vi "Construct DMD Intensity Coefficients (SubVI).vi"(7 "DMD #":enum16{"DMD1", "DMD2"}(ring), 8 "Number of Rows Processed":refnum<vi>, 11 "Image Size in":T1={"Height"=3072, "Width"=3200}) -> ()   [LabVIEW 2015]
uses:
  Controls (HOST)/Image Size.ctl
  <vilib>/Utility/file.llb/Read Delimited Spreadsheet (DBL).vi
  <vilib>/imath/engines/lvmath2/RunTimeEngine/Managers/WorkSpace/UID Generator.vi
  <vilib>/imath/engines/lvmath2/RunTimeEngine/RunTimeType/NIMS_RunTimeType_From StrictType (excl LVString).vi
  <instcachedir>/0/NIMS_RunTimeType_From StrictType (excl LVString)_EB1C38A9BC5048DA9ABDA8F781E54D21.lvgen/NIMS_RunTimeType_From StrictType (excl LVString)_EB1C38A9BC5048DA9ABDA8F781E54D21_031.vi
  <vilib>/imath/engines/lvmath2/RunTimeEngine/Struct/NIMS_StructSetField.vi
  <vilib>/imath/engines/lvmath2/RunTimeEngine/Struct/NIMS_StructGetField.vi
  <vilib>/imath/engines/lvmath2/RunTimeEngine/RunTimeType/NIMS_RunTimeType_To Numeric.vi
  <instcachedir>/0/NIMS_RunTimeType_To Numeric_B134FEC7BFC54ED5998F4CFD2EE98288.lvgen/NIMS_RunTimeType_To Numeric_B134FEC7BFC54ED5998F4CFD2EE98288_008.vi
  <instcachedir>/0/NIMS_RunTimeType_From StrictType (excl LVString)_EB1C38A9BC5048DA9ABDA8F781E54D21.lvgen/NIMS_RunTimeType_From StrictType (excl LVString)_EB1C38A9BC5048DA9ABDA8F781E54D21_000.vi
  <vilib>/imath/engines/lvmath2/RunTimeEngine/LocalVariableDefStatement/MC_LocalVariableDefStatement_Display.vi
  <vilib>/imath/engines/lvmath2/RunTimeEngine/Managers/SymbolTable/Clear UID.vi
  <vilib>/imath/engines/lvmath2/RunTimeEngine/NodeEndStatement/NIMS_NodeEndStatement_Output.vi
  <instcachedir>/0/NIMS_NodeEndStatement_Output_53EC0D466D134D7ABD903AC30B43404B.lvgen/NIMS_NodeEndStatement_Output_53EC0D466D134D7ABD903AC30B43404B_001.vi
  <vilib>/imath/engines/lvmath2/RunTimeEngine/ErrorHandling/NIMS_Finalize Error.vi
  <vilib>/Utility/file.llb/Write Delimited Spreadsheet (DBL).vi
  <vilib>/imath/engines/lvmath2/RunTimeEngine/Managers/SymbolTable/NIMS_WorkSpace.lvlib
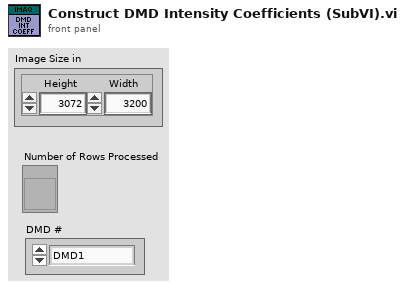
[diagram p1: front panel]
types:
  T1 = typedef "Image Size.ctl" = cluster{"Height":u16, "Width":u16}
  T2 = typedef "DMD 2 Calibration Parameters.ctl" = cluster{"xm1":dbl, "ym1":dbl, "xm2":dbl, "ym2":dbl, "xoff":dbl, "yoff":dbl}
  T3 = typedef "DMD 1 Calibration Parameters.ctl" = cluster{"xm1":dbl, "ym1":dbl, "xm2":dbl, "ym2":dbl, "xoff":dbl, "yoff":dbl}
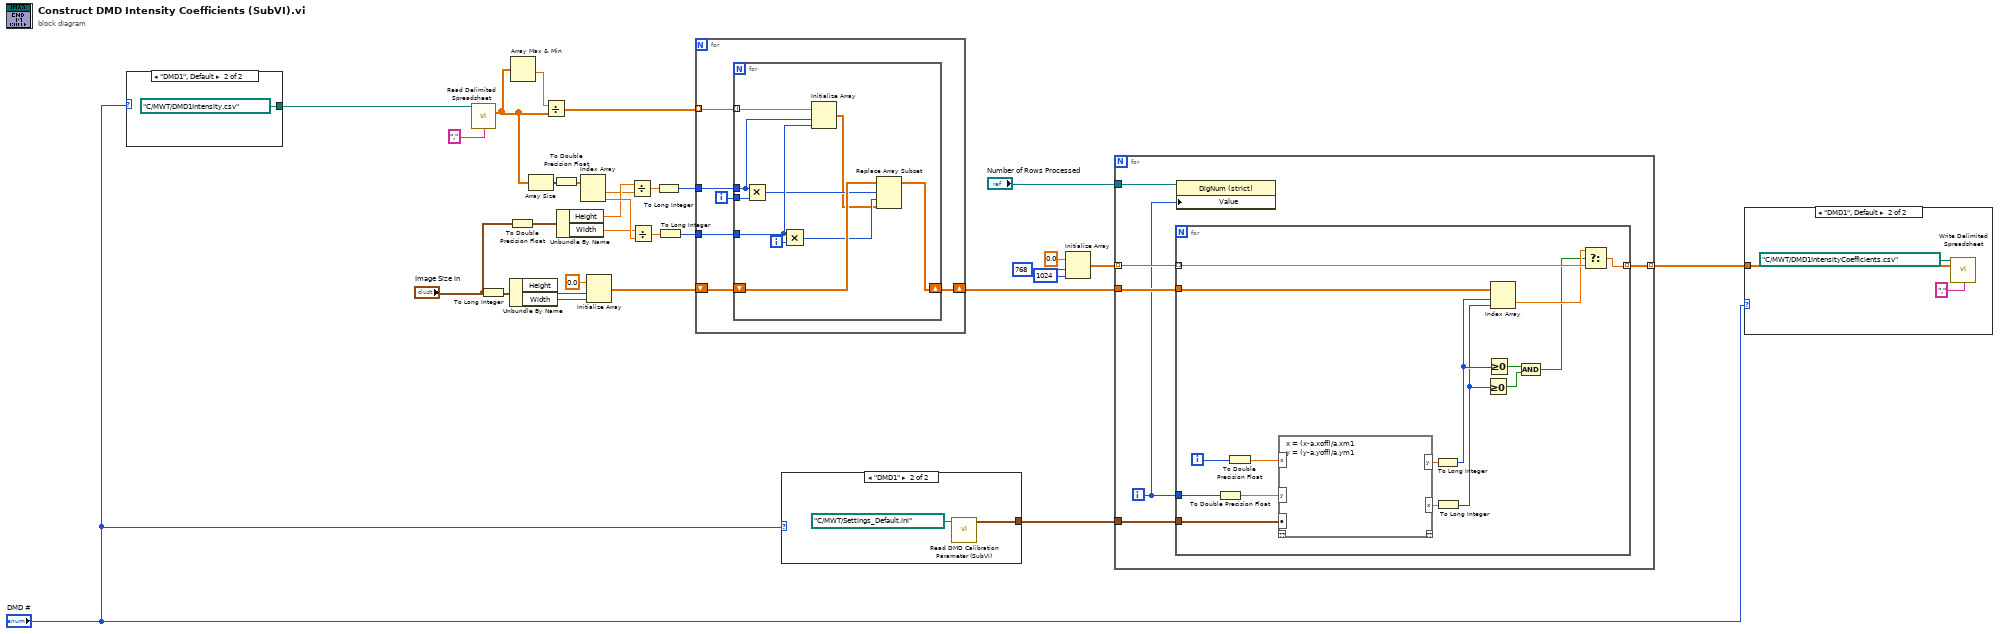
[diagram p0: block diagram]
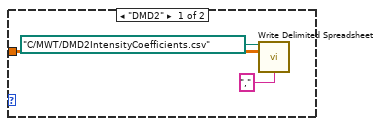
[diagram p2: hidden frame]
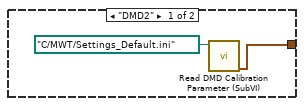
[diagram p3: hidden frame]
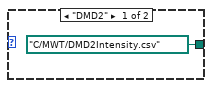
[diagram p4: hidden frame]
diagram:
  n1 = case shown="\"DMD1\", Default" "DMD #" {
    tunnel: [path "C:/MWT/DMD2Intensity.csv" ("file path (dialog if empty)") path "C:/MWT/DMD1Intensity.csv" ("file path (dialog if empty)")] -> w4
    frame "DMD2" {
    }
    frame "DMD1", Default {
    }
  }
  n2 = call-poly <vilib>:"Read Delimited Spreadsheet.vi"("file path (dialog if empty)"=w4, "delimiter (\\t)"="," ("delimiter (\\t)")) -> ("all rows"=w10:dbl[][])  [unwired: 8 in, 5 out]
  n3 = To Long Integer(number="Image Size in") -> (32bit integer=w9:cluster{"Height":i32, "Width":i32})
  n4 = To Double Precision Float(number="Image Size in") -> (double precision float=w15:cluster{"Height":dbl, "Width":dbl})
  n5 = Unbundle By Name(w9) -> ("Height"=w6:i32, "Width"=w7:i32)
  n6 = Array Max & Min(array=w10) -> (min value=w5:dbl)  [unwired: 3 out]
  n7 = Array Size(array=w10) -> (size(s)=w11:i32[])
  n8 = Divide(x=w5, y=w10) -> (x/y=w13:dbl[][])
  n9 = To Double Precision Float(number=w11) -> (double precision float=w14:dbl[])
  n10 = Unbundle By Name(w15) -> ("Height"=w17:dbl, "Width"=w18:dbl)
  n11 = Index Array(array=w14) -> (element #1=w16:dbl, element #2=w19:dbl)  [unwired: 2 in]
  n12 = Initialize Array(0.0 ("element"), w6, w7) -> (w12:dbl[][])
  n13 = Divide(x=w17, y=w16) -> (x/y=w20:dbl)
  n14 = Divide(x=w18, y=w19) -> (x/y=w21:dbl)
  n15 = To Long Integer(number=w20) -> (32bit integer=w22:i32)
  n16 = To Long Integer(number=w21) -> (32bit integer=w23:i32)
  n17 = for {
    shift-right: [w37] -> w25
    shift-left: w12 -> [w38]
    tunnel: w13 -> [w39] mode=indexing
    tunnel: w22 -> [w36]
    tunnel: w23 -> [w34]
    i -> [w35]
    n18 = for {
      tunnel: w39 -> [w45] mode=indexing
      shift-right: [w46] -> w37
      shift-left: w38 -> [w47]
      tunnel: w36 -> [w44]
      tunnel: w35 -> [w49]
      tunnel: w34 -> [w43]
      i -> [w48]
      n19 = Multiply(x=w44, y=w49) -> (x*y=w42:i32)
      n20 = Multiply(x=w43, y=w48) -> (x*y=w41:i32)
      n21 = Initialize Array(w45, w44, w43) -> (w40:dbl[][])
      n22 = Replace Array Subset(array=w47, new element=w40, index (row)=w42, index (col)=w41) -> (w46:dbl[][])
    }
  }
  n23 = case shown="\"DMD1\"" "DMD #" {
    tunnel: [w50 w53] -> w24
    frame "DMD2" {
      n24 = call "Read DMD Calibration Parameter (SubVI).vi"("Settings File Name"=path "C:/MWT/Settings_Default.ini") -> ("DMD 2 Calibration Parameters"=w50:T2)  [unwired: 9 in, 1 out]
    }
    frame "DMD1" {
      n25 = call "Read DMD Calibration Parameter (SubVI).vi"("Settings File Name"=path "C:/MWT/Settings_Default.ini") -> ("DMD 1 Calibration Parameters"=w53:T3)  [unwired: 9 in, 1 out]
    }
  }
  n26 = Initialize Array(0.0 ("element"), 768 ("dimension size"), 1024 ("dimension size")) -> (w29:dbl[][])
  n27 = for {
    tunnel: w24 -> [w58]
    tunnel: "Number of Rows Processed" -> [w56]
    tunnel: w25 -> [w57]
    tunnel: w29 -> [w59] mode=indexing
    tunnel: [w54] -> w2 mode=indexing
    i -> [w55]
    n28 = for {
      tunnel: w58 -> [w75]
      tunnel: w55 -> [w72]
      tunnel: w57 -> [w68]
      tunnel: w59 -> [w67] mode=indexing
      tunnel: [w66] -> w54 mode=indexing
      i -> [w74]
      n29 = To Double Precision Float(number=w72) -> (double precision float=w71:dbl)
      n30 = To Double Precision Float(number=w74) -> (double precision float=w73:dbl)
      n31 = mathscript code="x = (x-a.xoff)/a.xm1\ny = (y-a.yoff)/a.ym1"("x"=w73, "y"=w71, "a"=w75) -> ("y"=w70:dbl, "x"=w69:dbl)  [unwired: 1 in, 1 out]
      n32 = To Long Integer(number=w70) -> (32bit integer=w64:i32)
      n33 = To Long Integer(number=w69) -> (32bit integer=w63:i32)
      n34 = Greater Or Equal To 0?(x=w63) -> (x >= 0?=w61:bool)
      n35 = Greater Or Equal To 0?(x=w64) -> (x >= 0?=w62:bool)
      n36 = Index Array(array=w68, index (row)=w64, index (col)=w63) -> (element=w65:dbl)
      n37 = And(x=w62, y=w61) -> (x .and. y?=w60:bool)
      n38 = Select(t=w65, s=w60, f=w67) -> (s? t:f=w66:dbl)
    }
    n39 = property class="DigNum (strict)"(reference=w56, "Value"=w55) -> ()  [unwired: 1 in, 2 out]
  }
  n40 = case shown="\"DMD1\", Default" "DMD #" {
    tunnel: w2 -> [w182 w185]
    frame "DMD2" {
      n41 = call-poly <vilib>:"Write Delimited Spreadsheet.vi"("file path (dialog if empty)"=path "C:/MWT/DMD2IntensityCoefficients.csv", "2D data"=w182, "delimiter (\\t)"="," ("delimiter (\\t)")) -> ()  [unwired: 11 in, 2 out]
    }
    frame "DMD1", Default {
      n42 = call-poly <vilib>:"Write Delimited Spreadsheet.vi"("file path (dialog if empty)"=path "C:/MWT/DMD1IntensityCoefficients.csv", "2D data"=w185, "delimiter (\\t)"="," ("delimiter (\\t)")) -> ()  [unwired: 11 in, 2 out]
    }
  }
